vi "NewFocus Set Velocity and Acceleration.vi"(7 "Motion Settings":T1, 8 "error in (no error)":errorcluster, 9 "Device Address In":i32, 10 "DeviceKey In":string, 11 "CmdLib In":refnum<k24>) -> (0 "error out":errorcluster)   [LabVIEW 2021, in "NewFocus.lvclass"]
uses:
  NewFocus.lvclass
  C:/Development/prime/Prime-RIMAS/Focus/PicoMotor/CmdLib.dll
  PicoMotor/CmdLib.dll
  Focus cluster Motion Settings.ctl
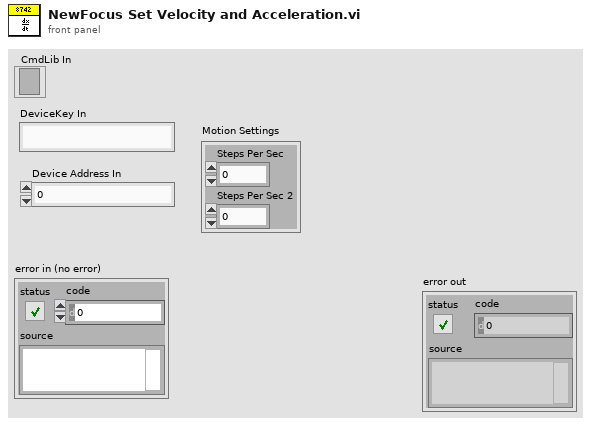
[diagram p1: front panel]
types:
  T1 = typedef "Focus cluster Motion Settings.ctl" = cluster{"Steps Per Sec":i32, "Steps Per Sec 2":i32}
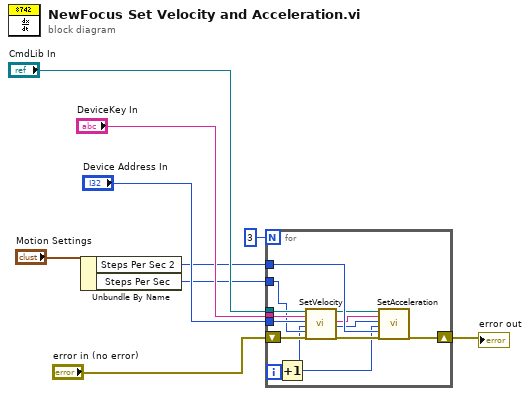
[diagram p0: block diagram]
diagram:
  n1 = Unbundle By Name("Motion Settings") -> ("Steps Per Sec 2"=w2:i32, "Steps Per Sec"=w3:i32)
  n2 = for {
    N: 3 -> [_]
    tunnel: "CmdLib In" -> [w19]
    tunnel: "DeviceKey In" -> [w18]
    tunnel: "Device Address In" -> [w17]
    shift-right: [w20] -> w8
    shift-left: "error in (no error)" -> [w22]
    tunnel: w3 -> [w16]
    tunnel: w2 -> [w15]
    i -> [w14]
    n3 = Increment(x=w14) -> (x+1=w10:i32)
    n4 = call "SetVelocity.vi"("CmdLib In"=w19, "DeviceKey In"=w18, "Device Address In"=w17, "Motor"=w10, "Steps Per Sec"=w16, "error in (no error)"=w22) -> ("CmdLib Out"=w11:refnum<k24>, "DeviceKey Out"=w12:string, "Device Address Out"=w13:i32, "error out"=w21:errorcluster)  [unwired: 10 in]
    n5 = call "SetAcceleration.vi"("CmdLib In"=w11, "DeviceKey In"=w12, "Device Address In"=w13, "Motor"=w10, "Steps Per Sec 2"=w15, "error in (no error)"=w21) -> ("error out"=w20:errorcluster)  [unwired: 10 in, 3 out]
  }
  "error out" <- w8
